vi "1 to 3 Up_movement(15pix).vi"(1 "Input pixmap":u8[][](array[numeric]), 2 "start Column":i32) -> (3 "Total point":i32, 4 "From:finish Col.":i32, 5 "moveLog(Row, Col.)":i32[][](array[numeric]), 6 "TapN":dbl)   [LabVIEW 2016]
panel:
  out "x-1":i32
  out "RupPoint":dbl[](array[numeric]) format="%_3f"
  out "startpoint":u8
  out "pointLog":i32[](array[numeric])
  out "3×3 point array":u8[][][](array[numeric])
  out "min. root p.":u8
  out "1forward":u8[](array[numeric])
  out "2forward":u8[](array[numeric])
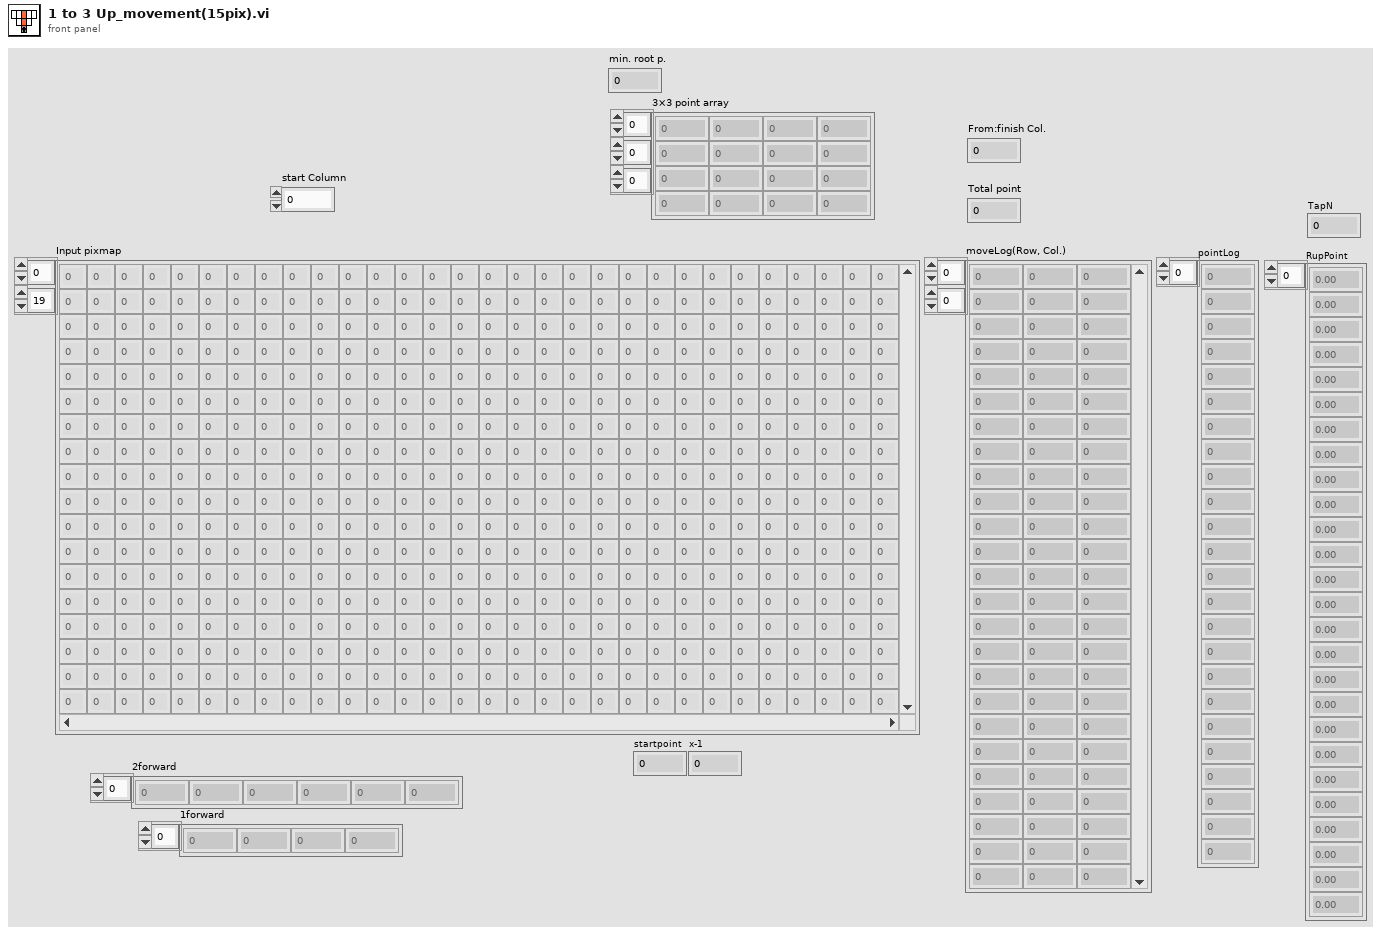
[diagram p1: front panel]
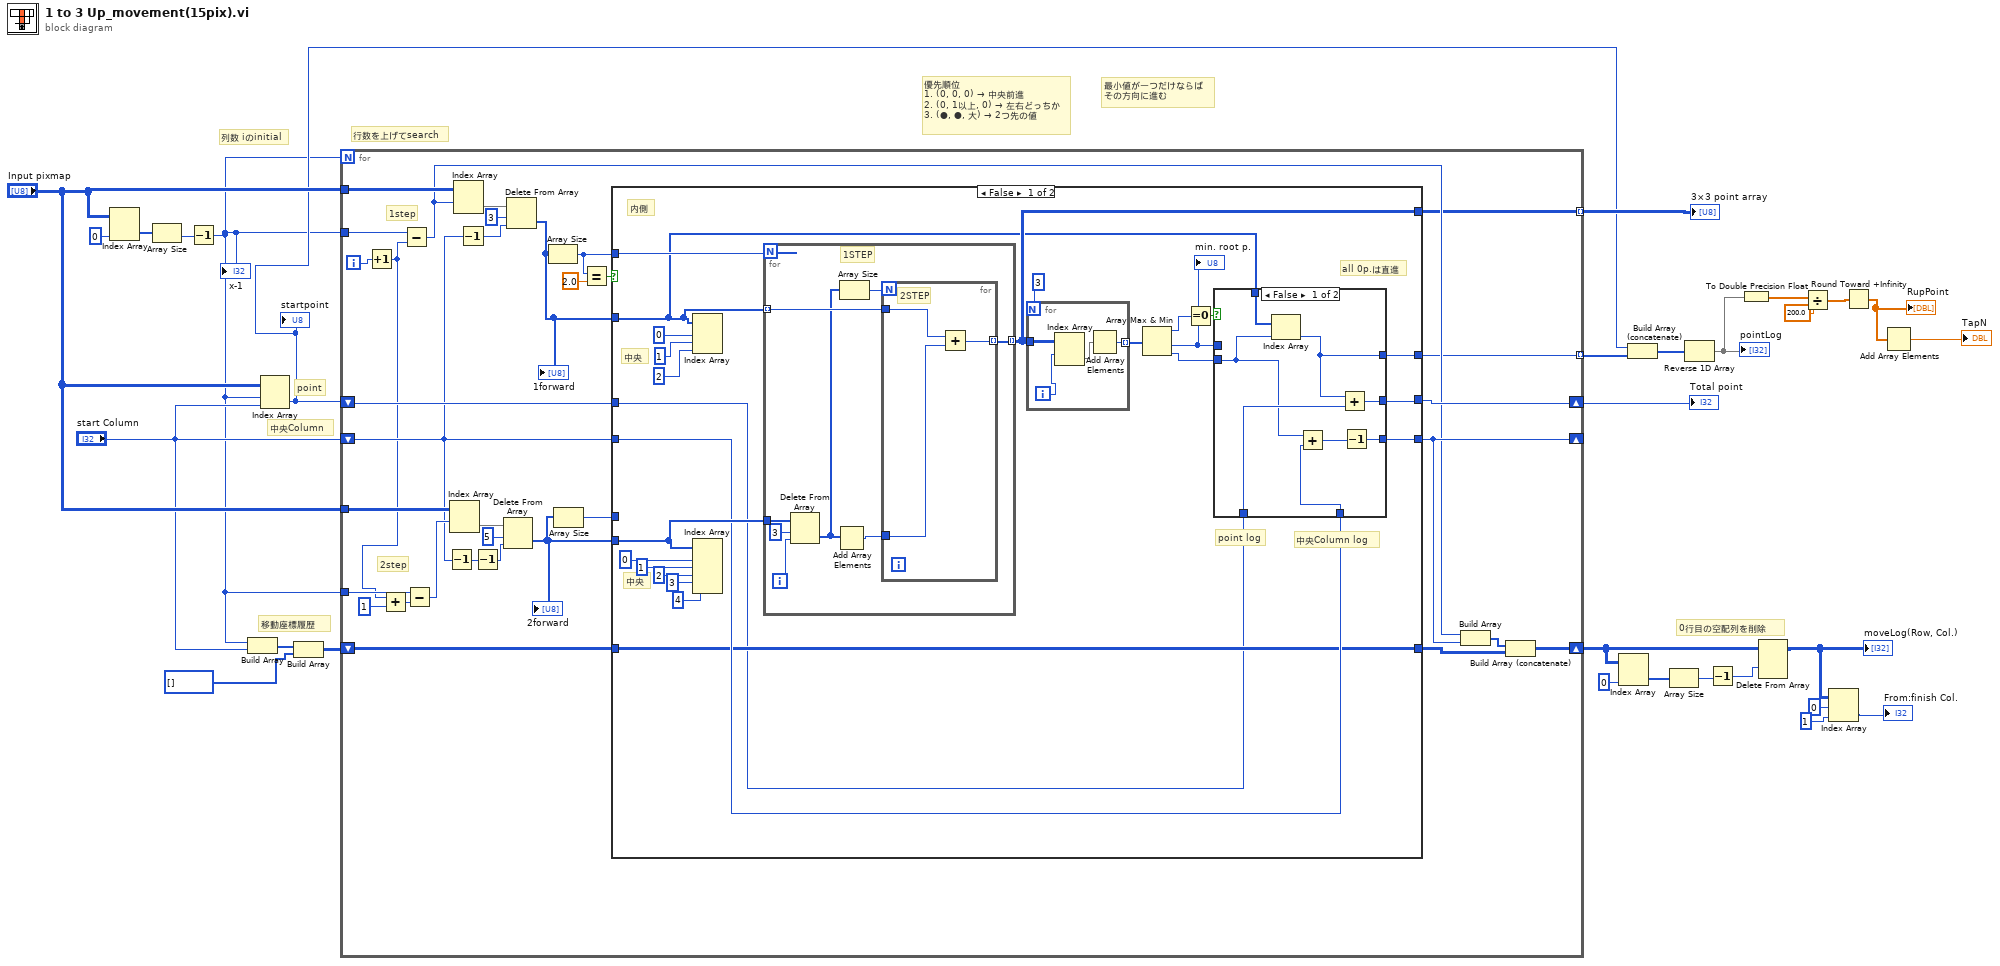
[diagram p0: block diagram]
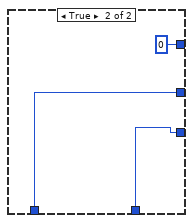
[diagram p2: hidden frame]
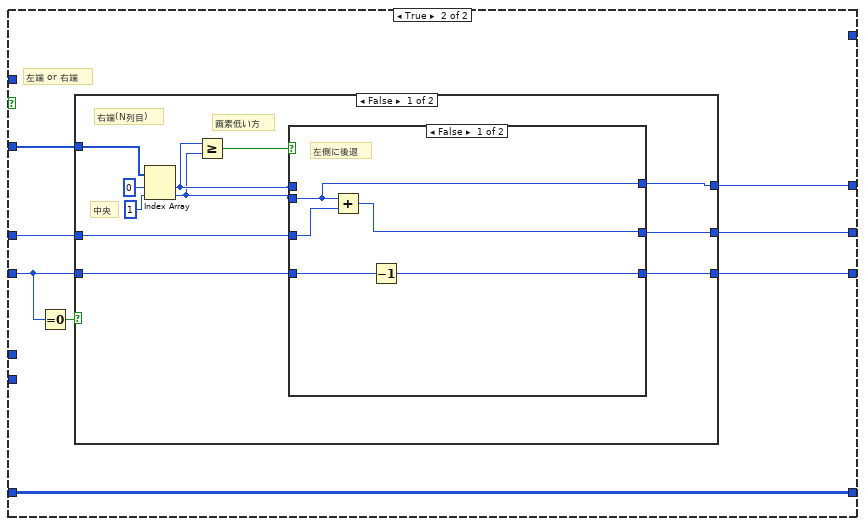
[diagram p3: hidden frame]
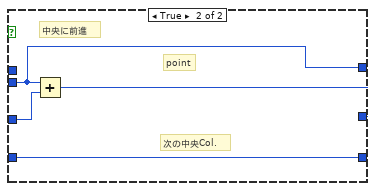
[diagram p4: hidden frame]
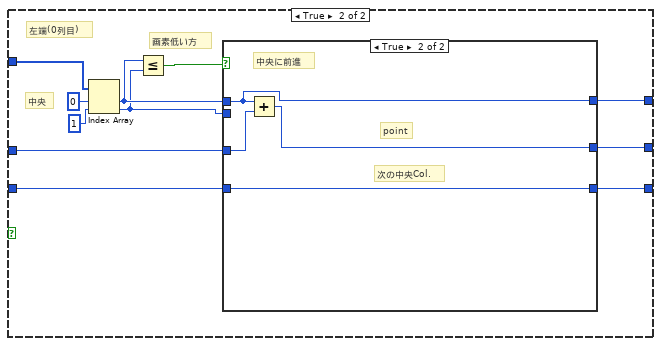
[diagram p5: hidden frame]
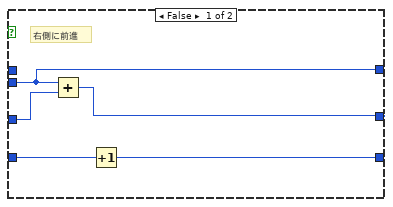
[diagram p6: hidden frame]
diagram:
  # "最小値が一つだけならば\nその方向に進む"
  # "優先順位\n1. (0, 0, 0) → 中央前進\n2. (0, 1以上, 0) → 左右どっちか\n3. (●, ●, 大) → 2つ先の値"
  # "0行目の空配列を削除"
  # "移動座標履歴"
  # "中央Column"
  # "point"
  # "行数を上げてsearch"
  # "列数 iのinitial"
  n1 = Index Array(array="Input pixmap", index (col)=0 ("無効な指標 （列）")) -> (element=w27:u8[])  [unwired: 1 in]
  n2 = Array Size(array=w27) -> (size(s)=w2:i32)
  n3 = Decrement(x=w2) -> (x-1=w1:i32)
  "x-1" <- w1
  n4 = Build Array(w1, "start Column") -> (w23:i32[])
  n5 = Index Array(array="Input pixmap", index (row)=w1, index (col)="start Column") -> (element=w11:u8)
  "startpoint" <- w11
  n6 = Build Array(w23, i32[] [] ("要素")) -> (w26:i32[][])
  n7 = for {
    N: w1 -> [_]
    tunnel: "Input pixmap" -> [w62]
    tunnel: w1 -> [w61]
    shift-right: [w53] -> w29
    shift-left: w11 -> [w54]
    shift-right: [w52] -> _
    shift-left: "start Column" -> [w39]
    shift-right: [w49] -> w18
    shift-left: w26 -> [w51]
    tunnel: "Input pixmap" -> [w44]
    tunnel: w1 -> [w38]
    tunnel: [w34] -> w24 mode=indexing
    tunnel: [w31] -> w10 mode=indexing
    i -> [w47]
    # "2step"
    # "1step"
    n8 = Increment(x=w47) -> (x+1=w30:i32)
    n9 = Add(x=w30, y=1) -> (x+y=w46:i32)
    n10 = Subtract(x=w61, y=w30) -> (x-y=w50:i32)
    n11 = Subtract(x=w38, y=w46) -> (x-y=w43:i32)
    n12 = Decrement(x=w39) -> (x-1=w40:i32)
    n13 = Index Array(array=w44, index (row)=w43) -> (element=w42:u8[])  [unwired: 1 in]
    n14 = Index Array(array=w62, index (row)=w50) -> (element=w60:u8[])  [unwired: 1 in]
    n15 = Decrement(x=w39) -> (x-1=w58:i32)
    n16 = Decrement(x=w40) -> (x-1=w41:i32)
    n17 = Delete From Array(array=w42, length=5 ("長さ"), index=w41) -> (deleted portion=w36:u8[])  [unwired: 1 out]
    "2forward" <- w36
    n18 = Delete From Array(array=w60, length=3 ("長さ"), index=w58) -> (deleted portion=w55:u8[])  [unwired: 1 out]
    "1forward" <- w55
    n19 = Array Size(array=w55) -> (size(s)=w37:i32)
    n20 = Array Size(array=w36) -> (size(s)=w35:i32)
    n21 = Equal?(x=w37, y=2.0) -> (x = y?=w56:bool)
    n22 = case shown="False" w56 {
      tunnel: w55 -> [w63 w120]
      tunnel: w54 -> [w65 w119]
      tunnel: [w76 w118] -> w53
      tunnel: w39 -> [w73 w115]
      tunnel: [w74 w117] -> w52
      tunnel: [w72 w114] -> w32
      tunnel: w51 -> [w72 w114]
      tunnel: w36 -> [w78 _]
      tunnel: w37 -> [w77 _]
      tunnel: w35 -> [_ _]
      tunnel: [w67 _] -> w34
      tunnel: [w64 w113] -> w31
      frame False {
        # "中央Column log"
        # "point log"
        # "all 0p.は直進"
        # "中央"
        # "中央"
        # "内側"
        n23 = Index Array(array=w63, index #1=0 ("指標"), index #2=1 ("指標"), index #3=2 ("指標")) -> ()  [unwired: 3 out]
        n24 = Index Array(array=w78, index #1=0 ("指標"), index #2=1 ("指標"), index #3=2 ("指標"), index #4=3 ("指標"), index #5=4 ("指標")) -> ()  [unwired: 5 out]
        n25 = for {
          N: w77 -> [_]
          tunnel: w63 -> [w109] mode=indexing
          tunnel: w78 -> [w107]
          tunnel: [w108] -> w67 mode=indexing
          i -> [w105]
          # "1STEP"
          n26 = Delete From Array(array=w107, length=3 ("長さ"), index=w105) -> (deleted portion=w103:u8[])  [unwired: 1 out]
          n27 = Add Array Elements(numeric array=w103) -> (sum=w102:u8)
          n28 = Array Size(array=w103) -> (size(s)=w104:i32)
          n29 = for {
            N: w104 -> [_]
            tunnel: w109 -> [w112]
            tunnel: [w111] -> w108 mode=indexing
            tunnel: w102 -> [w110]
            # "2STEP"
            n30 = Add(x=w112, y=w110) -> (x+y=w111:u8)
          }
        }
        n31 = for {
          N: 3 -> [_]
          tunnel: w67 -> [w87]
          tunnel: [w90] -> w68 mode=indexing
          i -> [w88]
          n32 = Index Array(array=w87, index (row)=w88) -> (element=w89:u8[])  [unwired: 1 in]
          n33 = Add Array Elements(numeric array=w89) -> (sum=w90:u8)
        }
        n34 = Array Max & Min(array=w68) -> (max value=w71:u8, min value=w69:u8, min index (indices)=w75:i32)  [unwired: 1 out]
        "min. root p." <- w69
        n35 = Equal To 0?(x=w71) -> (x = 0?=w70:bool)
        n36 = case shown="False" w70 {
          tunnel: w69 -> [_ _]
          tunnel: w65 -> [w98 w100]
          tunnel: [w97 w100] -> w76
          tunnel: w75 -> [w93 _]
          tunnel: [w96 w101] -> w74
          tunnel: w73 -> [w94 w101]
          tunnel: [w91 u8 0] -> w64
          tunnel: w63 -> [w92 _]
          frame False {
            n37 = Index Array(array=w92, index=w93) -> (element=w91:u8)
            n38 = Add(x=w93, y=w94) -> (x+y=w95:i32)
            n39 = Add(x=w91, y=w98) -> (x+y=w97:u8)
            n40 = Decrement(x=w95) -> (x-1=w96:i32)
          }
          frame True {
          }
        }
      }
      frame True {
        # "左端 or 右端"
        n41 = Equal To 0?(x=w115) -> (x = 0?=w116:bool)
        n42 = case shown="False" w116 {
          tunnel: w120 -> [w129 w151]
          tunnel: w119 -> [w125 w148]
          tunnel: [w123 w147] -> w118
          tunnel: w115 -> [w124 w146]
          tunnel: [w122 w145] -> w117
          tunnel: [w121 w141] -> w113
          frame False {
            # "中央"
            # "画素低い方"
            # "右端(N列目)"
            n43 = Index Array(array=w129, index #1=0 ("指標"), index #2=1 ("指標")) -> (element #1=w127:u8, element #2=w126:u8)
            n44 = Greater Or Equal?(x=w127, y=w126) -> (x >= y?=w128:bool)
            n45 = case shown="False" w128 {
              tunnel: w127 -> [_ _]
              tunnel: w125 -> [w133 w140]
              tunnel: [w136 w139] -> w123
              tunnel: w124 -> [w135 w138]
              tunnel: [w134 w138] -> w122
              tunnel: w126 -> [w132 w137]
              tunnel: [w132 w137] -> w121
              frame False {
                # "左側に後退"
                n46 = Add(x=w132, y=w133) -> (x+y=w136:u8)
                n47 = Decrement(x=w135) -> (x-1=w134:i32)
              }
              frame True {
                # "中央に前進"
                # "次の中央Col."
                # "point"
                n48 = Add(x=w137, y=w140) -> (x+y=w139:u8)
              }
            }
          }
          frame True {
            # "中央"
            # "画素低い方"
            # "左端(0列目)"
            n49 = Index Array(array=w151, index #1=0 ("指標"), index #2=1 ("指標")) -> (element #1=w143:u8, element #2=w142:u8)
            n50 = Less Or Equal?(x=w143, y=w142) -> (x <= y?=w144:bool)
            n51 = case shown="True" w144 {
              tunnel: w143 -> [_ w157]
              tunnel: w148 -> [w156 w160]
              tunnel: [w155 w159] -> w147
              tunnel: w146 -> [w154 w158]
              tunnel: [w153 w158] -> w145
              tunnel: w142 -> [w152 _]
              tunnel: [w152 w157] -> w141
              frame False {
                # "右側に前進"
                n52 = Add(x=w152, y=w156) -> (x+y=w155:u8)
                n53 = Increment(x=w154) -> (x+1=w153:i32)
              }
              frame True {
                # "中央に前進"
                # "次の中央Col."
                # "point"
                n54 = Add(x=w157, y=w160) -> (x+y=w159:u8)
              }
            }
          }
        }
      }
    }
    n55 = Build Array(w50, w52) -> (w33:i32[])
    n56 = Build Array (concatenate)(w33, w32) -> (w49:i32[][])
  }
  "Total point" <- w29
  "3×3 point array" <- w24
  n57 = Index Array(array=w18, index (col)=0 ("無効な指標 （列）")) -> (element=w20:i32[])  [unwired: 1 in]
  n58 = Build Array (concatenate)(w11, w10) -> (w9:u8[])
  n59 = Array Size(array=w20) -> (size(s)=w19:i32)
  n60 = Reverse 1D Array(array=w9) -> (reversed array=w8:u8[])
  "pointLog" <- w8
  n61 = Decrement(x=w19) -> (x-1=w17:i32)
  n62 = To Double Precision Float(number=w8) -> (double precision float=w7:dbl[])
  n63 = Delete From Array(array=w18, index (row)=w17) -> (array with subset deleted=w16:i32[][])  [unwired: 2 in, 1 out]
  "moveLog(Row, Col.)" <- w16
  n64 = Divide(x=w7, y=200.0) -> (x/y=w5:dbl[])
  n65 = Index Array(array=w16, index (row)=0 ("無効な指標 （行）"), index (col)=1 ("指標 （行）")) -> (element=→"From:finish Col.":i32)
  n66 = Round Toward +Infinity(x=w5) -> (ceil(x): smallest int >= x=w4:dbl[])
  "RupPoint" <- w4
  n67 = Add Array Elements(numeric array=w4) -> (sum=→"TapN":dbl)
